vi "Facade.vi"(0 "Data In":T4, 2 "Display State In":T2, 3 "Container State":T3) -> (6 "Data Out":T4, 7 "Display State Out":T2, 8 "Action":T1)   [LabVIEW 2019, in "ExpandHorizontal.xctl"]
uses:
  ExpandHorizontal.xctl
  Data.ctl
  <vilib>/_xctls/Container State.ctl
  State.ctl
  <vilib>/_xctls/Action.ctl
  <vilib>/_xctls/XControlSupport.lvlib
panel:
  in  "reSizeH":bool
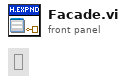
[diagram p1: front panel]
types:
  T1 = typedef "XControlSupport.lvlib/Action.ctl" = cluster{"Data Changed?":bool, "State Changed?":bool, "Action Name":string}
  T2 = typedef "ExpandHorizontal.xctl/State.ctl" = cluster{"Size":i16, "Expanded":bool}
  T3 = typedef "XControlSupport.lvlib/Container State.ctl" = cluster{"Indicator?":bool, "Run Mode?":bool, " Refnum":refnum<vi>}
  T4 = typedef "ExpandHorizontal.xctl/Data.ctl" = bool
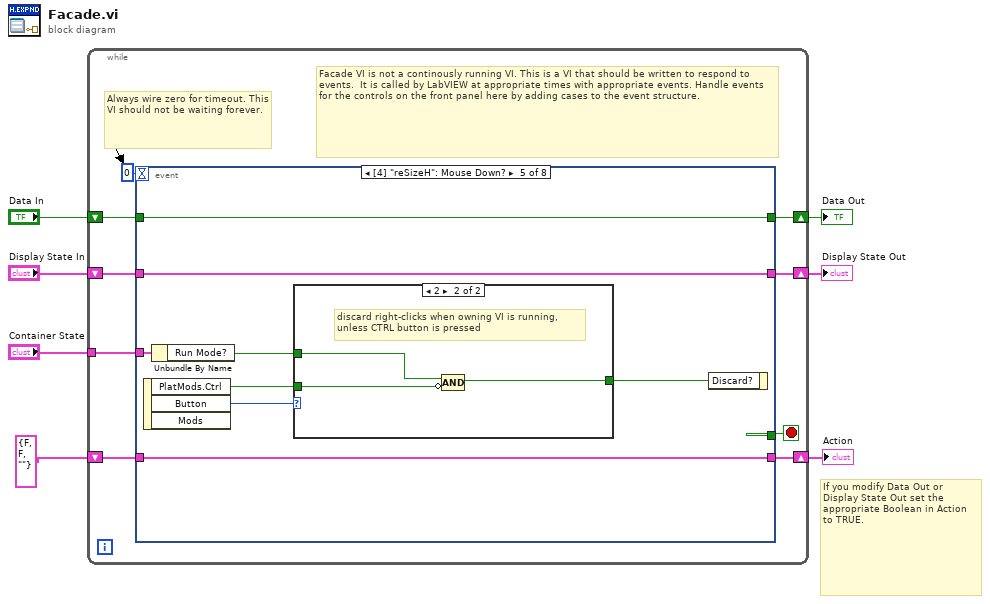
[diagram p0: block diagram]
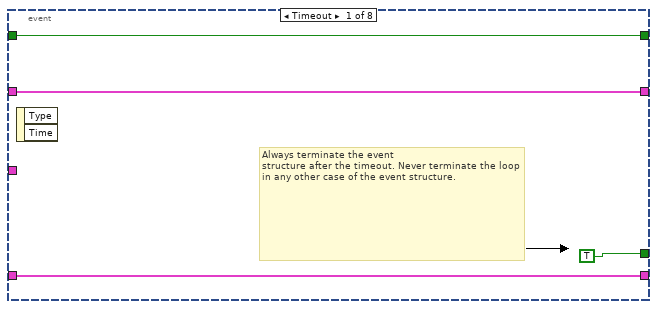
[diagram p2: hidden frame]
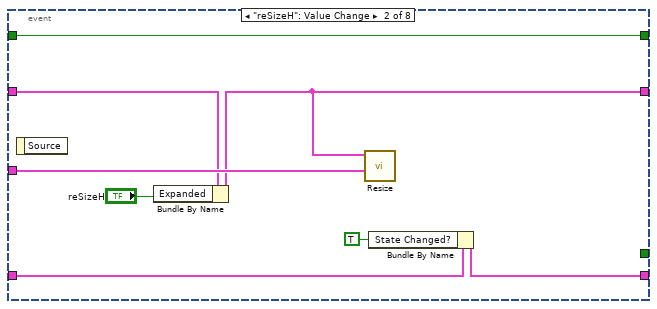
[diagram p3: hidden frame]
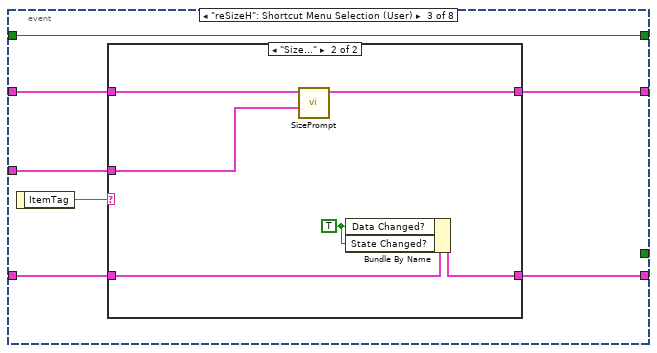
[diagram p4: hidden frame]
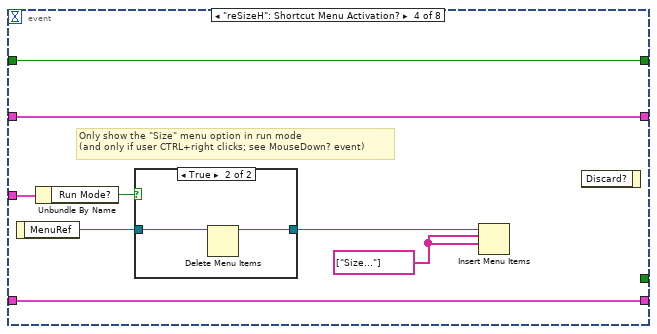
[diagram p6: hidden frame]
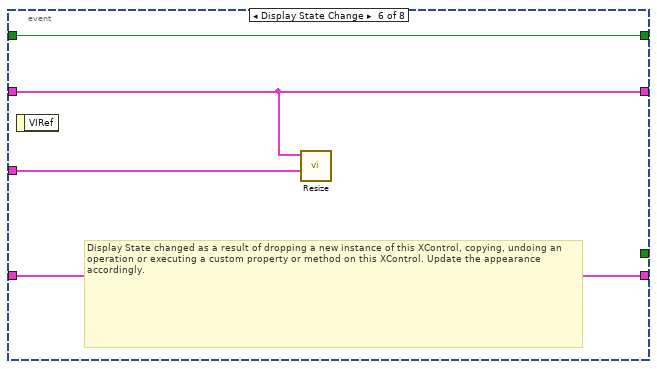
[diagram p9: hidden frame]
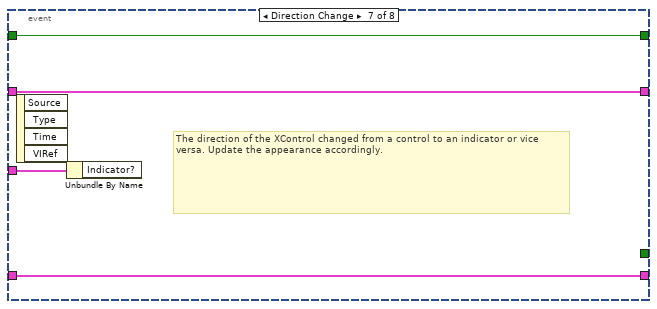
[diagram p10: hidden frame]
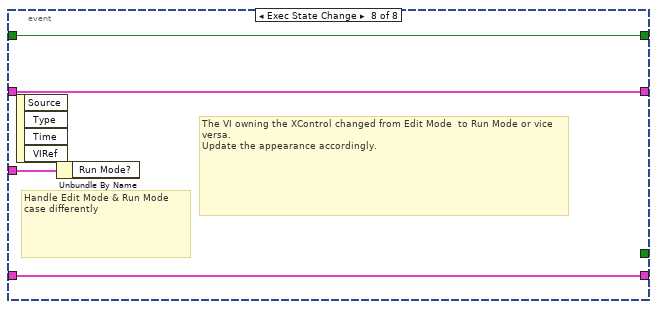
[diagram p11: hidden frame]
diagram:
  # "If you modify Data Out or\nDisplay State Out set the\nappropriate Boolean in Action\nto TRUE."
  n1 = while {
    shift-right: [w15] -> w4
    shift-left: "Display State In" -> [w16]
    tunnel: "Container State" -> [w12]
    shift-right: [w10] -> w7
    shift-left: "Data In" -> [w11]
    shift-right: [w8] -> w2
    shift-left: T1 {"Data Changed?"=FALSE, "State Changed?"=FALSE, "Action Name"=""} ("Action") -> [w9]
    stop <- w14 stop-if-true
    # "Facade VI is not a continously running VI. This is a VI that should be written to respond to events.  It is called by LabVIEW at appropriate times with appropriate events. Handle events for the controls on the front panel here by adding cases to the event structure."
    # "Always wire zero for timeout. This\nVI should not be waiting forever."
    n2 = event shown="[4] \"reSizeH\": Mouse Down?" {
      selector: _ -> [_ _ _ _ _ _ _ _]
      dyn-events: _ -> [_ _ _ _ _ _ _ _]
      timeout: 0 -> [_ _ _ _ _ _ _ _]
      tunnel: w16 -> [w18 w25 w33 w51 w62 w67 w72 w76]
      tunnel: [w18 w24 w32 w51 w62 w67 w72 w76] -> w15
      tunnel: [TRUE _ _ _ _ _ _ _] -> w14
      tunnel: w12 -> [_ w27 w29 w46 w55 w66 w73 w77]
      tunnel: w11 -> [w17 w28 w35 w50 w61 w69 w71 w75]
      tunnel: [w17 w28 w35 w50 w61 w69 w71 w75] -> w10
      tunnel: [w19 w22 w30 w49 w60 w68 w70 w74] -> w8
      tunnel: w9 -> [w19 w23 w31 w49 w60 w68 w70 w74]
      event Timeout {
        # "Always terminate the event\nstructure after the timeout. Never terminate the loop in any other case of the event structure."
        n3 = event-data() -> ()  [unwired: 1 in, 2 out]
      }
      event "reSizeH": Value Change {
        n4 = event-data() -> ()  [unwired: 1 in, 1 out]
        n5 = Bundle By Name(cluster=w25, "Expanded"="reSizeH") -> (w24:T2)
        n6 = call "Resize.vi"("Container State"=w27, "Display State In"=w24) -> ()  [unwired: 10 in]
        n7 = Bundle By Name(cluster=w23, "State Changed?"=TRUE) -> (w22:T1)
      }
      event "reSizeH": Shortcut Menu Selection (User) {
        n8 = event-data() -> ("ItemTag"=w34:string)  [unwired: 1 in]
        n9 = case shown="\"Size...\"" w34 {
          tunnel: w33 -> [w37 w43]
          tunnel: [w37 w42] -> w32
          tunnel: w31 -> [w36 w41]
          tunnel: [w36 w39] -> w30
          tunnel: w29 -> [_ w40]
          frame Default {
          }
          frame "Size..." {
            w38 = TRUE ("Data Changed?")
            n10 = call "SizePrompt.vi"("Container State"=w40, "Display State In in"=w43) -> ("Display State In out"=w42:T2)  [unwired: 9 in]
            n11 = Bundle By Name(cluster=w41, "Data Changed?"=w38, "State Changed?"=w38) -> (w39:T1)
          }
        }
      }
      event "reSizeH": Shortcut Menu Activation? {
        w47 = string[] ["Size..."] ("item names")
        # "Only show the \"Size\" menu option in run mode\n(and only if user CTRL+right clicks; see MouseDown? event)"
        n12 = event-data() -> ("MenuRef"=w48:refnum<k9>)  [unwired: 1 in]
        n13 = Unbundle By Name(w46) -> ("Run Mode?"=w44:bool)
        n14 = case shown="True" w44 {
          tunnel: w48 -> [w52 w54]
          tunnel: [w52 w53] -> w45
          frame False {
          }
          frame True {
            n15 = Delete Menu Items(9:w54) -> (3:w53:refnum<k9>)  [unwired: 3 in, 1 out]
          }
        }
        n16 = Insert Menu Items(7:w47, 8:w47, 9:w45) -> ()  [unwired: 3 in, 3 out]
        n17 = event-data() -> ()  [unwired: 2 in, 1 out]
      }
      event "reSizeH": Mouse Down? {
        n18 = event-data() -> ("PlatMods.Ctrl"=w57:bool, "Button"=w58:u16)  [unwired: 1 in, 1 out]
        n19 = Unbundle By Name(w55) -> ("Run Mode?"=w56:bool)
        n20 = case shown="2" w58 {
          tunnel: [_ w65] -> w59
          tunnel: w57 -> [_ w64]
          tunnel: w56 -> [_ w63]
          frame 0, Default {
          }
          frame 2 {
            # "discard right-clicks when owning VI is running,\nunless CTRL button is pressed"
            n21 = Compound Arithmetic op=AND(w63, invert w64) -> (w65:bool)
          }
        }
        n22 = event-data("Discard?"=w59) -> ()  [unwired: 1 in, 1 out]
      }
      event Display State Change {
        # "Display State changed as a result of dropping a new instance of this XControl, copying, undoing an operation or executing a custom property or method on this XControl. Update the appearance accordingly."
        n23 = event-data() -> ()  [unwired: 1 in, 1 out]
        n24 = call "Resize.vi"("Container State"=w66, "Display State In"=w67) -> ()  [unwired: 10 in]
      }
      event Direction Change {
        # "The direction of the XControl changed from a control to an indicator or vice versa. Update the appearance accordingly."
        n25 = event-data() -> ()  [unwired: 1 in, 4 out]
        n26 = Unbundle By Name(w73) -> ()  [unwired: 1 out]
      }
      event Exec State Change {
        # "The VI owning the XControl changed from Edit Mode  to Run Mode or vice versa.\nUpdate the appearance accordingly."
        # "Handle Edit Mode & Run Mode\ncase differently"
        n27 = event-data() -> ()  [unwired: 1 in, 4 out]
        n28 = Unbundle By Name(w77) -> ()  [unwired: 1 out]
      }
    }
  }
  "Display State Out" <- w4
  "Data Out" <- w7
  "Action" <- w2
